vi "ATF-DO Data display.vi"(11 "DO":waveform(dbl)[](array[waveform])) -> ()   [LabVIEW 2022 SP3]
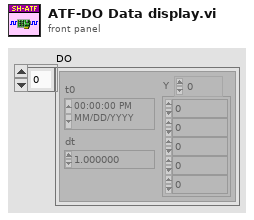
[diagram p1: front panel]
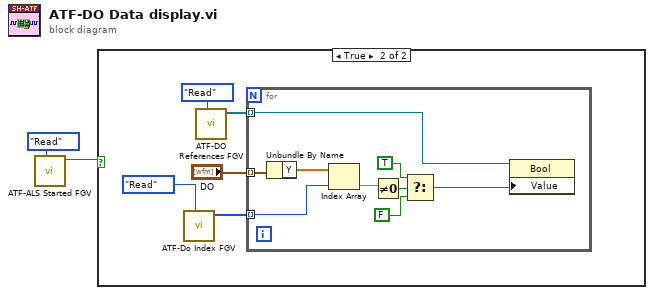
[diagram p0: block diagram]
diagram:
  n1 = call "ATF-ALS Started FGV.vi"("Enum"=enum16{"Read", "Write"}."Read") -> ("Als started R"=w1:bool)  [unwired: 9 in, 1 out]
  n2 = case shown="True" w1 {
    frame False {
    }
    frame True {
      n3 = call "ATF-Do Index FGV.vi"("State"=enum16{"Write", "Read"}."Read") -> ("Storage index"=w4:i32[])  [unwired: 9 in, 1 out]
      n4 = call "ATF-DO References FGV.vi"("State"=enum16{"Init", "Read", "Write"}."Read") -> ("DO ref out"=w5:refnum<vi>[])  [unwired: 9 in, 1 out]
      n5 = for {
        tunnel: "DO" -> [w16] mode=indexing
        tunnel: w5 -> [w9] mode=indexing
        tunnel: w4 -> [w10] mode=indexing
        n6 = Unbundle By Name(w16) -> ("Y"=w15:dbl[])
        n7 = Index Array(array=w15, index=w10) -> (element=w13:dbl)
        n8 = Not Equal To 0?(x=w13) -> (x != 0?=w14:bool)
        n9 = Select(t=TRUE, s=w14, f=FALSE) -> (s? t:f=w8:bool)
        n10 = property class="Bool"(reference=w9, "Value"=w8) -> ()  [unwired: 1 in, 2 out]
      }
    }
  }
